vi "Main Test App.vi"() -> ()   [LabVIEW 2011]
panel:
  out "Limit Test Passed?":bool
  in  "Lower LED Limit (V)":dbl=1.63
  in  "Upper LED Limit (V)":dbl=1.635
  out "LED Test Passed?":bool
  in  "Filter Error Limits (+/- V)":dbl=0.06
  out "Limit Test Results":cluster{dbl[], dbl[]}[](graph)=[{[1000.0, 9166.666666666668, 17333.333333333336, 25500.0, 33666.66666666667, 41833.333333333336, 50000.0], [0.8109999999999999, 0.7375, 0.6639999999999999, 0.5905, 0.5169999999999999, 0.44349999999999995, 0.37]}, {[1000.0, 9166.666666666668, 17333.333333333336, 25500.0, 33666.66666666667, 41833.333333333336, 50000.0], [0.7794851199823166, 0.7105386097097423, 0.600359382509452, 0.5104585406834482, 0.4415120304108739, 0.3921679593334433, 0.3549909194805846]}, {[1000.0, 9166.666666666668, 17333.333333333336, 25500.0, 33666.66666666667, 41833.333333333336, 50000.0], [0.6910000000000001, 0.6174999999999999, 0.544, 0.4705, 0.39699999999999996, 0.32349999999999995, 0.25]}]
  in  "Select XML Config File":u16(ring)=2 items=["PXI Mod Instr Config 081226.xml", "Legacy Instr Config 081226.xml", "Simulated Instruments.xml"]
  out "Actual LED Voltage (V)":dbl
  in  "error in (no error)":errorcluster
  out "error out":errorcluster
  in  "Number of Steps":i32=7
  in  "Start Frequency (>1K Hz)":dbl=1000.0
  in  "Stop Frquency (<50k Hz)":dbl=50000.0
  # "Filter Limit Test Results"
  # "Filter Limit Test Parameters"
  # "LED Test Parameters"
  # "LED Test Results"
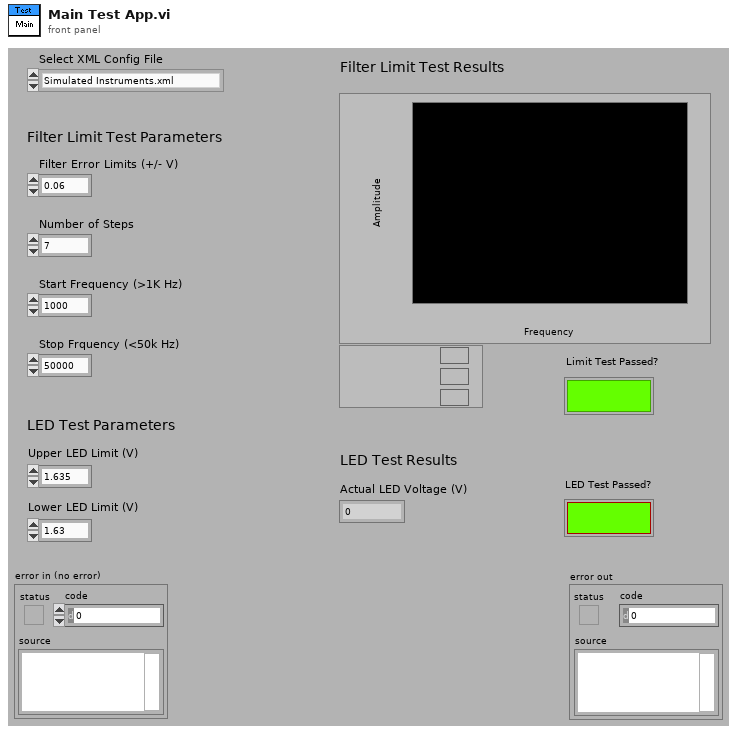
[diagram p1: front panel]
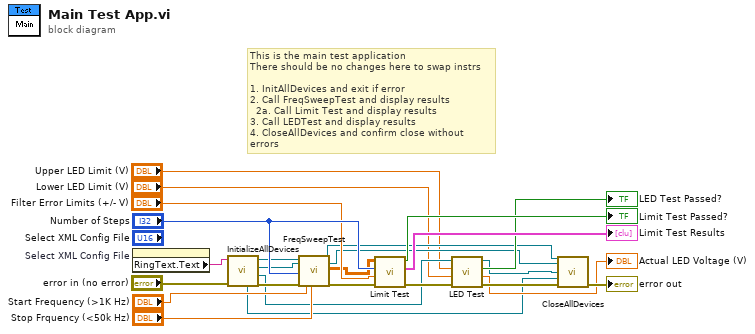
[diagram p0: block diagram]
diagram:
  # "This is the main test application\nThere should be no changes here to swap instrs\n\n1. InitAllDevices and exit if error\n2. Call FreqSweepTest and display results\n  2a. Call Limit Test and display results\n3. Call LEDTest and display results\n4. CloseAllDevices and confirm close without errors"
  n1 = property on="Select XML Config File" class="Ring (strict)"() -> ("RingText.Text"=w4:string)  [unwired: 2 in, 2 out]
  n2 = call "InitializeAllDevices.vi"("error in (no error)"="error in (no error)", "XML File Name"=w4) -> ("error out"=w13:errorcluster, "Meter"=w10:refnum<class "Meter.lvclass">, "Scope"=w14:refnum<class "Scope.lvclass">, "Signal Generator"=w15:refnum<class "Signal Generation.lvclass">, "Switch"=w3:refnum<class "Switch.lvclass">)  [unwired: 5 in]
  n3 = call "FreqSweepTest.vi"("Signal Generator"=w15, "Scope"=w14, "Number of Steps (25)"="Number of Steps", "error in (no error)"=w13, "Start Frequency (1000)"="Start Frequency (>1K Hz)", "Stop Frequency (50000)"="Stop Frquency (<50k Hz)") -> ("Signal Generator Out"=w8:refnum<class "Signal Generation.lvclass">, "Scope Out"=w7:refnum<class "Scope.lvclass">, "Freq Amp Array"=w6:dbl[][], "error out"=w23:errorcluster)  [unwired: 10 in]
  n4 = call "Limit Test.vi"("error in (no error)"=w23, "Filter Error Limits"="Filter Error Limits (+/- V)", "Number of Steps"="Number of Steps", "Freq Amp Array"=w6) -> ("error out"=w17:errorcluster, "Limit Test Results"=→"Limit Test Results":cluster{dbl[], dbl[]}[], "Test Passed?"=→"Limit Test Passed?":bool)  [unwired: 1 in, 4 out]
  n5 = call "LED Test.vi"("error in (no error)"=w17, "Lower LED Limit (V)"="Lower LED Limit (V)", "Upper LED Limit (V)"="Upper LED Limit (V)", "Meter"=w10) -> ("error out"=w24:errorcluster, "Diode Voltage"=→"Actual LED Voltage (V)":dbl, "LED Test Passed?"=→"LED Test Passed?":bool, "Meter Out"=w9:refnum<class "Meter.lvclass">)  [unwired: 4 out]
  n6 = call "CloseAllDevices.vi"("Signal Generator"=w8, "Scope"=w7, "Meter"=w9, "Switch"=w3, "error in (no error)"=w24) -> ("error out"=→"error out":errorcluster)  [unwired: 10 in]
